vi "Write Supported Protocols.vi"(8 "error in (no error)":errorcluster, 10 "Supported Protocols":string[](array[string]), 11 "Connection.WS in":refnum<class "Connection.WS.lvclass">) -> (0 "error out":errorcluster, 3 "Connection.WS out":refnum<class "Connection.WS.lvclass">)   [LabVIEW 2013, in "Connection.WS_GOSPL.lvlib" / "Connection.WS.lvclass"]
uses:
  Connection.WS.lvclass
  Connection.WS.lvclass/Connection.WS.ctl
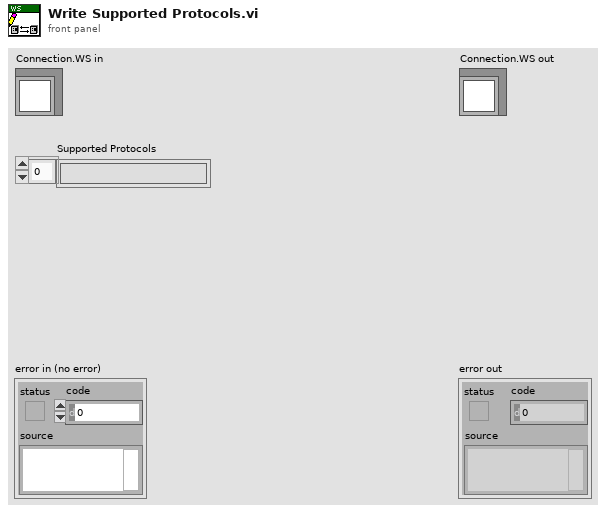
[diagram p1: front panel]
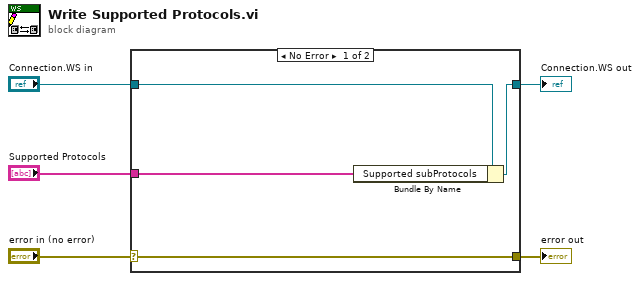
[diagram p0: block diagram]
diagram:
  n1 = case shown="No Error" "error in (no error)" {
    selector: "error in (no error)" -> [w9 w10]
    tunnel: [w9 w10] -> w4
    tunnel: [w7 w11] -> w2
    tunnel: "Connection.WS in" -> [w8 w11]
    tunnel: "Supported Protocols" -> [w6 _]
    frame No Error {
      n2 = Bundle By Name(cluster=w8, "Supported subProtocols"=w6) -> (w7:refnum<class "Connection.WS.lvclass">)
    }
    frame Error {
    }
  }
  "error out" <- w4
  "Connection.WS out" <- w2
